vi "GetPrimaryIPaddress.vi"(8 "error in (no error)":errorcluster, 11 "Network Adapter Settings":T1[](array[typedef]) {"IP Address Request Mode" items=["Static"=1, "DHCP/Link Local"=2, "Link-Local Only"=4, "DHCP Only"=8]; "Adapter Mode" items=["Disabled"=1, "TCP/IP Ethernet"=2, "Deterministic"=4, "EtherCAT"=8, "TCP/IP WLAN Connect"=32, "TCP/IP WLAN Create"=64]}) -> (0 "error out":errorcluster, 3 "primary ip address":string)   [LabVIEW 2017, in "USBDrive.lvlib"]
uses:
  <vilib>/addons/InsightCM/Devices/Shared/Common/USBDrive/USBDrive.lvlib
  <vilib>/addons/SystemInfoProcess/controls/NetworkAdapterSettings.ctl
  <vilib>/addons/SystemInfoProcess/SystemInfoProcess.lvlib
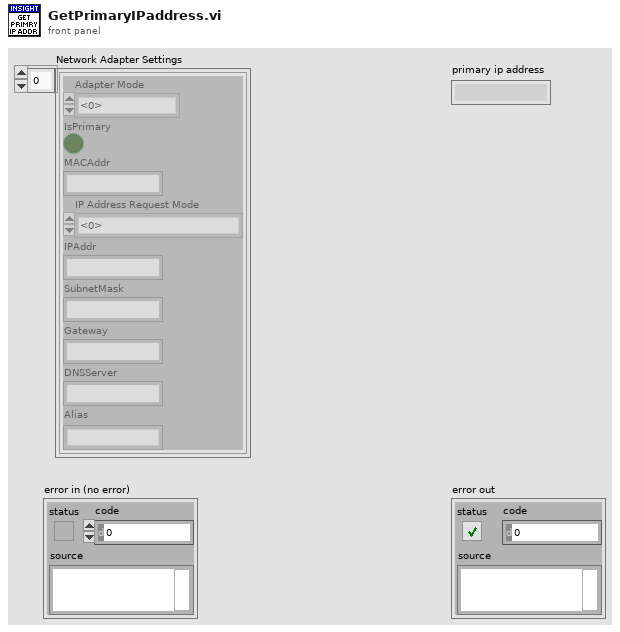
[diagram p1: front panel]
types:
  T1 = typedef "SystemInfoProcess.lvlib/NetworkAdapterSettings.ctl" = cluster{"Adapter Mode":u32, "IsPrimary":bool, "MACAddr":string, "IP Address Request Mode":u32, "IPAddr":string, "SubnetMask":string, "Gateway":string, "DNSServer":string, "Alias":string}
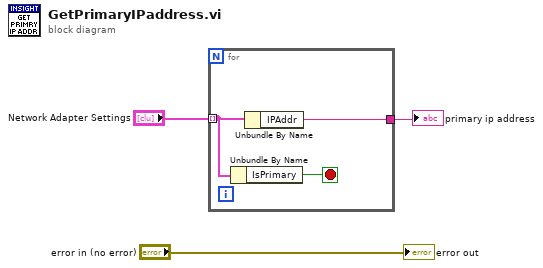
[diagram p0: block diagram]
diagram:
  n1 = for {
    tunnel: "Network Adapter Settings" -> [w5] mode=indexing
    tunnel: [w4] -> w1
    stop <- w6 stop-if-true
    n2 = Unbundle By Name(w5) -> ("IsPrimary"=w6:bool)
    n3 = Unbundle By Name(w5) -> ("IPAddr"=w4:string)
  }
  "primary ip address" <- w1
  "error out" <- "error in (no error)"
